vi "TraverseControl_High.vi"(0 "Mode":T2=enum."Read traverse position", 1 "Route Checking?":bool, 2 "Home":T1, 3 "Traverse Name":string, 7 "Model       Roll      Pitch       Yaw (deg)":sgl[](array[numeric]) format="%#.2f", 11 "Position input XYZ":sgl[](array[numeric])=[0.0, 0.0, 0.0] format="%.2f", 12 "Last Part of Move?":bool, 13 "Speed Factor":sgl=1.0 min=0.1 max=5 format="%.2f", 14 "Backlash Compensation?":bool=TRUE) -> (4 "Position Output XYZ":sgl[](array[numeric]) format="%.2f", 15 "Error String":string)   [LabVIEW 2015]
uses:
  Anemometry/Anemometry Sub Vis/Gen Trav/Trav_mode.ctl
  Anemometry/Anemometry Sub Vis/Controls/Home.ctl
  Anemometry/Anemometry Sub Vis/Globals/Trav_pos_global.vi
  Anemometry/Anemometry Sub Vis/Gen Trav/Route mapping/Route_mapping_global.vi
  Anemometry/Anemometry Sub Vis/Globals/Preference_global.vi
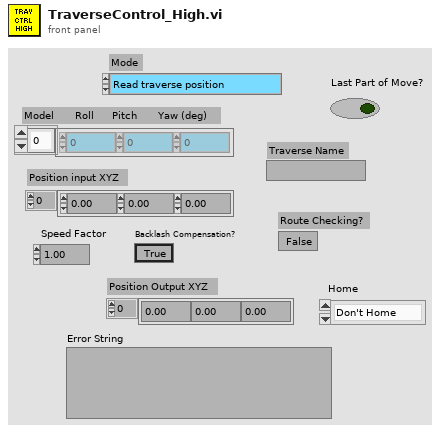
[diagram p1: front panel]
types:
  T1 = typedef "Home.ctl" = enum16{"Don't Home", "Home  +X", "Home  -X", "Home  +Y", "Home  -Y", "Home  +Z", "Home  -Z"}
  T2 = typedef "Trav_mode.ctl" = enum16{"Move traverse", "Read traverse position", "Teach Position"}
  T3 = typedef "Tunnel_Coordinates.ctl" = enum16{"Work in Tunnel Coordinates", "Work in Model Coordinates"}
  T4 = typedef "Box_size.ctl" = cluster{"Max":sgl, "Min":sgl}[]
  T5 = typedef "Exclude_cluster.ctl" = cluster{"Sizes":T4, "Name":string, "Exclude Type":T6}
  T6 = typedef "Exclusion_type.ctl" = enum16{"Exclude completely", "Allow only vertical moves"}
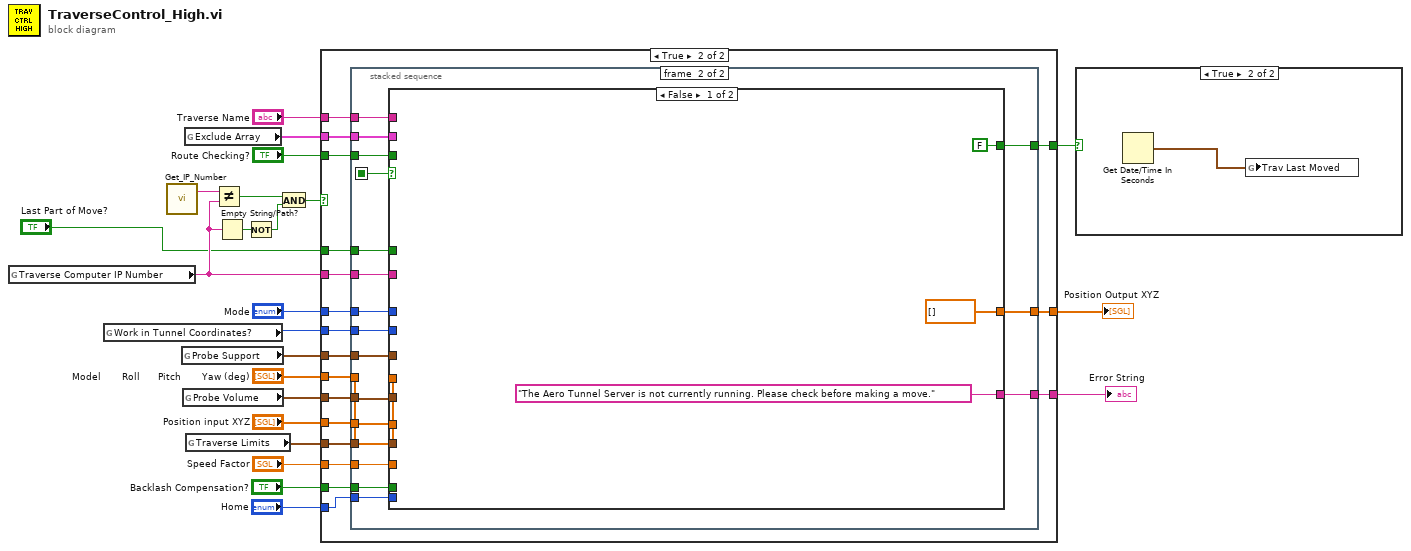
[diagram p0: block diagram]
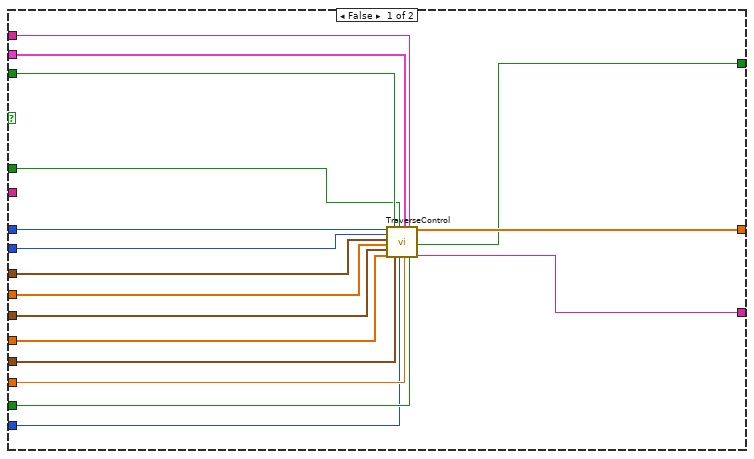
[diagram p3: hidden frame]
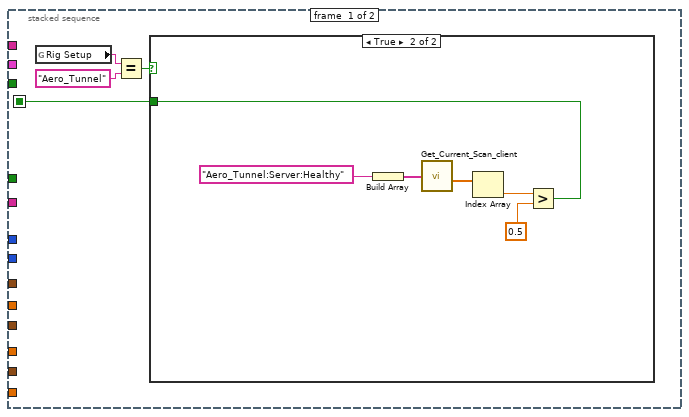
[diagram p4: hidden frame]
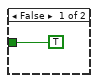
[diagram p5: hidden frame]
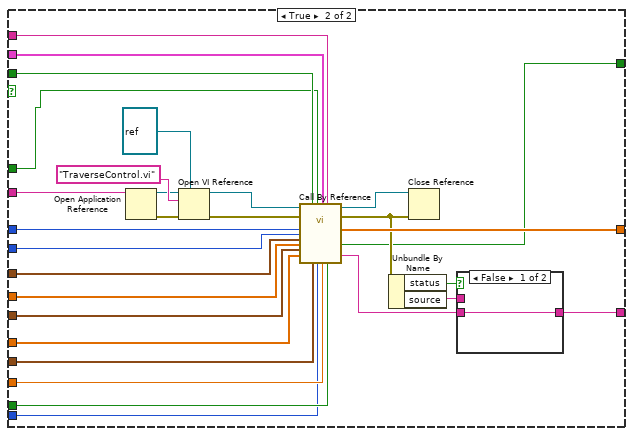
[diagram p6: hidden frame]
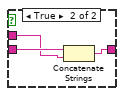
[diagram p7: hidden frame]
diagram:
  n1 = global read "Trav_pos_global.vi" "Traverse Computer IP Number"() -> (w11:string)
  n2 = global read "Trav_pos_global.vi" "Work in Tunnel Coordinates?"() -> (w5:T3)
  n3 = call "Get_IP_Number.vi"() -> ("IP Number"=w23:string)  [unwired: 1 out]
  n4 = global read "Route_mapping_global.vi" "Probe Support"() -> (w4:T4)
  n5 = global read "Route_mapping_global.vi" "Probe Volume"() -> (w6:T4)
  n6 = global read "Route_mapping_global.vi" "Exclude Array"() -> (w8:T5[])
  n7 = global read "Route_mapping_global.vi" "Traverse Limits"() -> (w7:T4)
  n8 = Not Equal?(x=w23, y=w11) -> (x != y?=w10:bool)
  n9 = Empty String/Path?(string/path=w11) -> (empty?=w13:bool)
  n10 = Not(x=w13) -> (.not. x?=w12:bool)
  n11 = And(x=w10, y=w12) -> (x .and. y?=w9:bool)
  n12 = case shown="True" w9 {
    tunnel: "Route Checking?" -> [w33 w58]
    tunnel: "Traverse Name" -> [w32 w57]
    tunnel: [w39 w56] -> w20
    tunnel: [w40 w48] -> w19
    tunnel: "Backlash Compensation?" -> [w36 w55]
    tunnel: "Speed Factor" -> [w35 w54]
    tunnel: "Position input XYZ" -> [w38 w53]
    tunnel: "Model       Roll      Pitch       Yaw (deg)" -> [w37 w52]
    tunnel: "Mode" -> [w34 w51]
    tunnel: w11 -> [_ w50]
    tunnel: w8 -> [w31 w49]
    tunnel: w7 -> [w30 w45]
    tunnel: w6 -> [w29 w46]
    tunnel: w5 -> [w28 w47]
    tunnel: w4 -> [w27 w44]
    tunnel: "Last Part of Move?" -> [w26 w43]
    tunnel: "Home" -> [w25 w42]
    tunnel: [w24 w41] -> w1
    frame False {
      n13 = call "TraverseControl.vi"("Mode"=w34, "Work in Tunnel Coordinates?"=w28, "Probe Support"=w27, "Model       Roll      Pitch       Yaw (deg)"=w37, "Probe Volume"=w29, "Position input XYZ"=w38, "Route Checking?"=w33, "Entire Space"=w30, "Last Part of Move?"=w26, "Home"=w25, "Exclude Array"=w31, "Speed Factor"=w35, "Traverse Name"=w32, "Backlash Compensation?"=w36) -> ("Position Output XYZ"=w39:sgl[], "Moved?"=w24:bool, "Error String"=w40:string)  [unwired: 3 in]
    }
    frame True {
      n14 = stacked-sequence {
        seq-local: [w59 _] -> [_ w74]
        tunnel: w58 -> [_ w88]
        tunnel: w57 -> [_ w87]
        tunnel: [_ w86] -> w56
        tunnel: w55 -> [_ w85]
        tunnel: w54 -> [_ w84]
        tunnel: w53 -> [_ w83]
        tunnel: w52 -> [_ w82]
        tunnel: w51 -> [_ w81]
        tunnel: w50 -> [_ w80]
        tunnel: w49 -> [_ w79]
        tunnel: [_ w78] -> w48
        tunnel: w47 -> [_ w77]
        tunnel: w46 -> [_ w76]
        tunnel: w45 -> [_ w75]
        tunnel: w44 -> [_ w73]
        tunnel: w43 -> [_ w72]
        tunnel: w42 -> [_ w71]
        tunnel: [_ w70] -> w41
        frame #0 {
          n15 = global read "Preference_global.vi" "Rig Setup"() -> (w62:string)
          n16 = Equal?(x=w62, y="Aero_Tunnel" ("Rig Setup")) -> (x = y?=w60:bool)
          n17 = case shown="True" w60 {
            tunnel: [TRUE w64] -> w59
            frame False {
            }
            frame True {
              n18 = Build Array("Aero_Tunnel:Server:Healthy") -> (w69:string[])
              n19 = call "Get_Current_Scan_client.vi"("ADAM Ch Names"=w69) -> ("Numerical Values"=w67:dbl[])  [unwired: 3 out]
              n20 = Index Array(array=w67) -> (element=w66:dbl)  [unwired: 1 in]
              n21 = Greater?(x=w66, y=0.5) -> (0:w64:bool)
            }
          }
        }
        frame #1 {
          n22 = case shown="False" w74 {
            tunnel: w88 -> [_ w117]
            tunnel: w87 -> [_ w116]
            tunnel: [sgl[] [] ("Position Output XYZ") w115] -> w86
            tunnel: w85 -> [_ w114]
            tunnel: w84 -> [_ w113]
            tunnel: w83 -> [_ w112]
            tunnel: w82 -> [_ w111]
            tunnel: w81 -> [_ w110]
            tunnel: w80 -> [_ w107]
            tunnel: w79 -> [_ w104]
            tunnel: ["The Aero Tunnel Server is not currently running. Please check before making a move." ("Error String") w101] -> w78
            tunnel: w77 -> [_ w98]
            tunnel: w76 -> [_ w97]
            tunnel: w75 -> [_ w96]
            tunnel: w73 -> [_ w95]
            tunnel: w72 -> [_ w94]
            tunnel: w71 -> [_ w93]
            tunnel: [FALSE ("Moved?") w92] -> w70
            frame False {
            }
            frame True {
              n23 = Open Application Reference(11:w107) -> (0:w105:errorcluster, 3:w106:refnum<vi>)  [unwired: 2 in, 1 out]
              n24 = Open VI Reference(type specifier VI Refnum (for type only)=refnum<vi> refnum ("Scout Server"), application reference (local)=w106, vi path="TraverseControl.vi", error in (no error)=w105) -> (vi reference=w118:refnum<vi>, error out=w109:errorcluster)  [unwired: 2 out]
              n25 = call-by-ref "?"(reference=w118, error in=w109, "Mode"=w110, "Work in Tunnel Coordinates?"=w98, "Probe Support"=w95, "Model       Roll      Pitch       Yaw (deg)"=w111, "Probe Volume"=w97, "Position input XYZ"=w112, "Route Checking?"=w117, "Entire Space"=w96, "Last Part of Move?"=w94, "Home"=w93, "Exclude Array"=w104, "Speed Factor"=w113, "Traverse Name"=w116, "Backlash Compensation?"=w114) -> (reference out=w108:refnum<vi>, error out=w103:errorcluster, "Position Output XYZ"=w115:sgl[], "Moved?"=w92:bool, "Error String"=w100:string)  [unwired: 3 in]
              n26 = Unbundle By Name(w103) -> ("status"=w102:bool, "source"=w99:string)
              n27 = Close Reference(reference=w108, error in (no error)=w103) -> ()  [unwired: 1 out]
              n28 = case shown="False" w102 {
                tunnel: [w121 w124] -> w101
                tunnel: w100 -> [w121 w123]
                tunnel: w99 -> [_ w122]
                frame False {
                }
                frame True {
                  n29 = Concatenate Strings(w123, w122) -> (w124:string)
                }
              }
            }
          }
        }
      }
    }
  }
  "Error String" <- w19
  "Position Output XYZ" <- w20
  n30 = case shown="True" w1 {
    frame False {
    }
    frame True {
      n31 = Get Date/Time In Seconds() -> (seconds since 1Jan1904=w125:timestamp)
      n32 = global write "Trav_pos_global.vi" "Trav Last Moved"(w125) -> ()
    }
  }
